vi "SaveDataFile.vi"(6 "Settings":T1={"Name of test"="", "Date"=timestamp(0 s since 1904-01-01), "Location"="", "Template"="", "Soundcard"="", "resolution"=32, "Sampling rate"=48000, "Ch1 Gain "=25.0, "Ch2 Gain"=10.0, "Sample time (s)"=0.3, "Pre-trigger (s)"=0.01, "Hammer Threshold"=10.0, "Positions"=12, "Taps/Position"=5, "Set Names"="", "Freq resolution"=10.0, "Hammer cutoff"=0.0, "Mic cutoff"=0.0, "Double bounce "=0.0, "Hammer Cal"=10.0, "dB Offset"=0.0, "Accel Cal"=10.0, "Vibrometer Cal"=0.0, "Mic Cal"=0.0, "Output"=2, "Voltage Cal"=1.0, "Vibrometer Port"="ASRL27::INSTR", "Range"=4, "High Pass"=2, "Bandwidth"=4, "X Range"=[], "Y Range"=[], "dB Spread"=0.0, "Trigger"=0, "Ch_1"=25, "Ch_2"=25, "flip?"=FALSE, "60Hz"=FALSE, "Time offset"=0.0, "Piezo Cal"=1.0, "Default Notes"=""} {"Ch_2" min=1 step=1; "Ch_1" min=1 max=100 step=1; "Trigger" items=["Hammer (force)", "Self-tap", "Spacebar"]; "Bandwidth" items=["1 kHz"=1, "5 kHz"=5, "10 kHz"=10, "25 kHz"=25, "50 kHz"=50, "100 kHz"=100]; "High Pass" items=["Off", "13 Hz", "104 Hz"]; "Range" items=["10 mm/s"=1, "20 mm/s"=2, "50 mm/s"=5, "100 mm/s"=10, "200 mm/s"=20, "500 mm/s"=50, "1 m/s"=100, "2 m/s"=200]; "Output" items=["Accelerometer", "Speed (from acceleration)", "Microphone", "Vibrometer", "Piezo"]; "Voltage Cal" format="%#_13g"; "Ch2 Gain" format="%#_13g"; "Ch1 Gain" format="%#_13g"; "Double bounce" min=0.0; "Mic cutoff" min=0.0 format="%#_4g"; "Hammer cutoff" min=0.0 format="%#_4g"; "Freq resolution" min=0.0; "Pre-trigger (s)" format="%#_13g"; "Date" format="%<%H:%M\n%d/%m/%y>T"; "resolution" items=["16 bit"=16, "24 bit"=24, "32 bit"=32]; "Sampling rate" items=["22050 samp/s"=22050, "44100 samp/s"=44100, "48000 samp/s"=48000]}, 7 "Alarms":refnum<vi>, 8 "error in (no error)":errorcluster, 11 "Data":waveform(dbl)[](array[waveform])) -> (0 "error out":errorcluster, 1 "last tap?":bool, 2 "New File?":bool, 3 "new path":path, 4 "Name of test":string)   [LabVIEW 2022 SP3]
uses:
  PreferencesControl.ctl
  Mic/Mic_Global.vi
panel:
  out "Alarms":string
  # "output, input"
  # "Hz"
  # "dB"
  # "dB"
  # "sec"
  # "sec"
  # "mV/Pa"
  # "mV/m/s2"
  # "mV/mm/s"
  # "V/N"
  # "sec"
  # "sec"
  # "mV/N"
  # "a.u."
  # "a.u."
  # "sec"
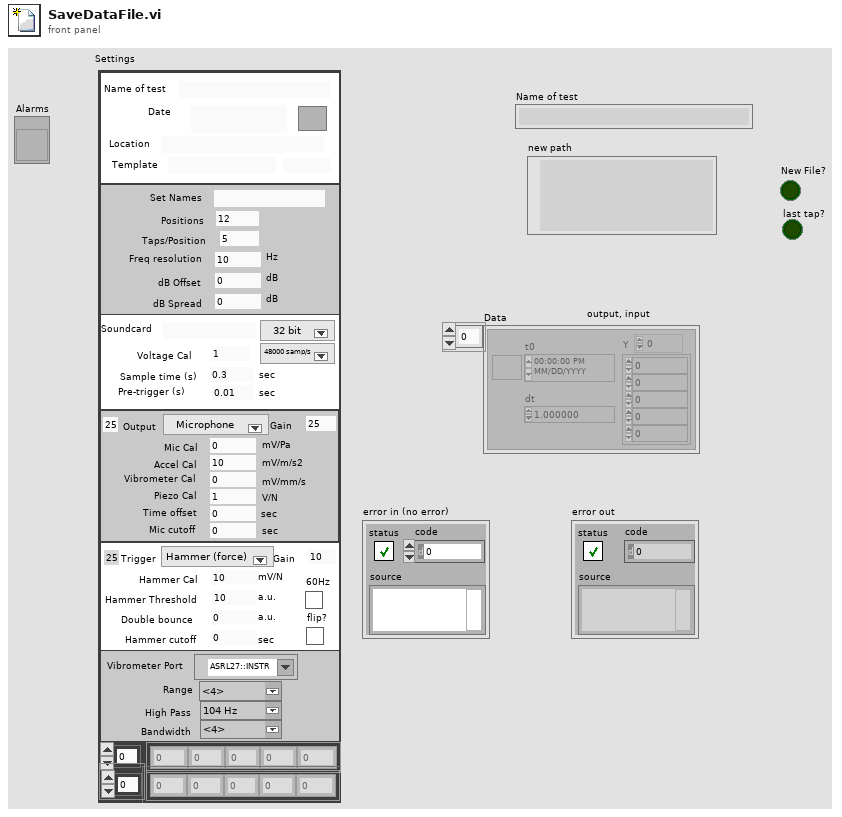
[diagram p1: front panel]
types:
  T1 = typedef "PreferencesControl.ctl" = cluster{"Name of test":string, "Date":timestamp, "Location":string, "Template":string, "Soundcard":string, "resolution":u16, "Sampling rate":u16, "Ch1 Gain ":dbl, "Ch2 Gain":dbl, "Sample time (s)":dbl, "Pre-trigger (s)":dbl, "Hammer Threshold":dbl, "Positions":i16, "Taps/Position":i16, "Set Names":string, "Freq resolution":dbl, "Hammer cutoff":dbl, "Mic cutoff":dbl, "Double bounce ":dbl, "Hammer Cal":dbl, "dB Offset":dbl, "Accel Cal":dbl, "Vibrometer Cal":dbl, "Mic Cal":dbl, "Output":u16, "Voltage Cal":dbl, "Vibrometer Port":refnum<visa-resource-name>, "Range":u16, "High Pass":u16, "Bandwidth":u16, "X Range":cluster{"Minimum":dbl, "Maximum":dbl, "Increment":dbl, "Minor Increment":dbl, "Start":dbl}[], "Y Range":cluster{"Minimum":dbl, "Maximum":dbl, "Increment":dbl, "Minor Increment":dbl, "Start":dbl}[], "dB Spread":dbl, "Trigger":u16, "Ch_1":u8, "Ch_2":u8, "flip?":bool, "60Hz":bool, "Time offset":dbl, "Piezo Cal":dbl, "Default Notes":string}
  T2 = cluster{"Alerts":bool, "Log X Axis":bool, "dB scale":bool, "Averaging":bool, "Fade":dbl, "Centroids?":bool}
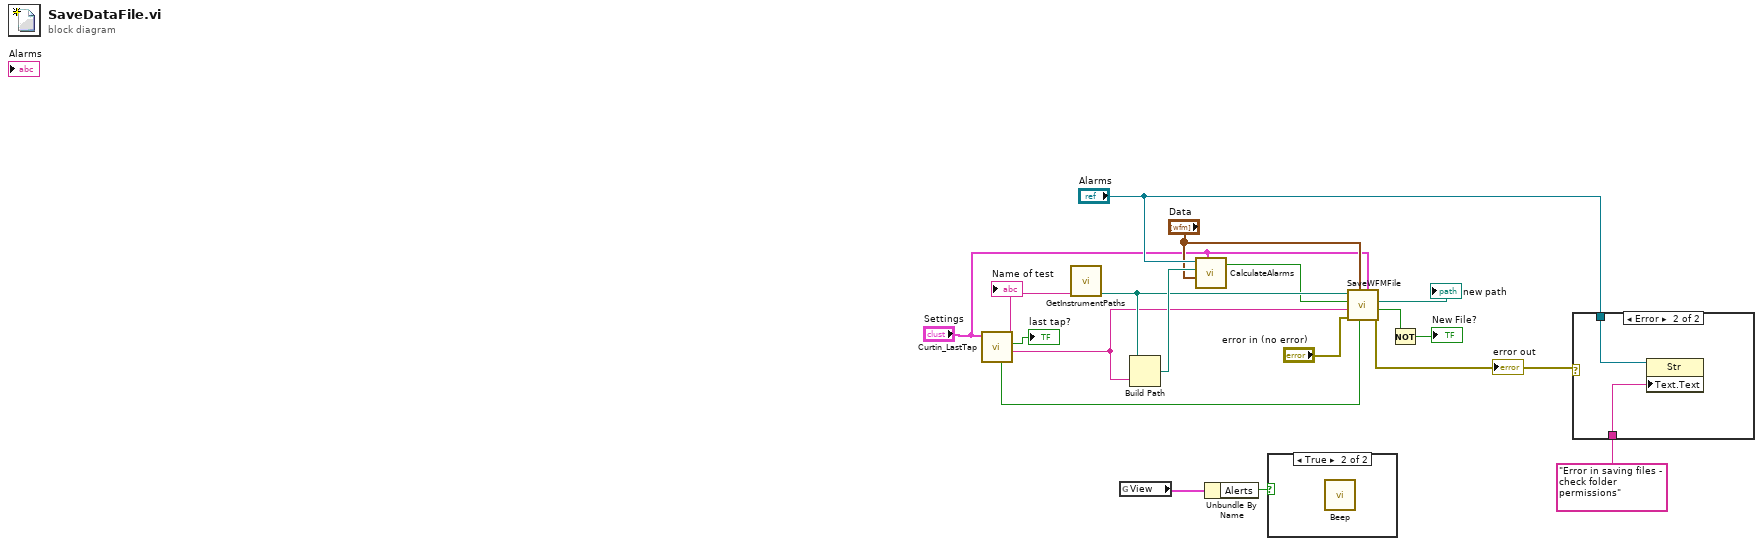
[diagram p0: block diagram]
diagram:
  n1 = call "Curtin_LastTap.vi"("Settings"="Settings") -> ("New File"=w8:string, "New position?"=→"last tap?":bool, "Name of test"=w18:string, "Done?"=w5:bool)  [unwired: 5 in, 2 out]
  "Name of test" <- w18
  n2 = call "GetInstrumentPaths.vi"("Instrument"=w18) -> ("Path To Raw Folder"=w10:path)  [unwired: 6 in, 4 out]
  n3 = global read "Mic_Global.vi" "View"() -> (w17:T2)
  n4 = Build Path(base path=w10, name or relative path=w8) -> (appended path=w11:path)
  n5 = call "CalculateAlarms.vi"("Settings"="Settings", "last tap"="Data", "Last Path"=w11, "Alarm"="Alarms") -> ("Good point?"=w9:bool)  [unwired: 6 in, 1 out]
  n6 = Unbundle By Name(w17) -> ("Alerts"=w16:bool)
  n7 = case shown="True" w16 {
    frame False {
    }
    frame True {
      n8 = call <vilib>:"Beep.vi"() -> ()  [unwired: 12 in]
    }
  }
  n9 = call "SaveWFMFile.vi"("Settings"="Settings", "Done? in"=w5, "Data"="Data", "error in (no error)"="error in (no error)", "New File"=w8, "Good point?"=w9, "Path To Raw Folder"=w10) -> ("error out"=w4:errorcluster, "Done? out"=w3:bool, "new file path"=→"new path":path)  [unwired: 1 in, 1 out]
  "error out" <- w4
  n10 = Not(x=w3) -> (.not. x?=→"New File?":bool)
  n11 = case shown="Error" w4 {
    tunnel: "Alarms" -> [_ w20]
    tunnel: "Error in saving files - check folder permissions" ("Alarms") -> [_ w19]
    frame No Error {
    }
    frame Error {
      n12 = property class="Str"(reference=w20, "Text.Text"=w19) -> ()  [unwired: 1 in, 2 out]
    }
  }
